vi "cRIO Open Module Detect_9104.vi"(8 "error in (no error)":errorcluster, 11 "RIO Device":string="RIO0") -> (0 "error out":errorcluster, 2 "slots":i32, 3 "Refnum out":refnum<k20>)   [LabVIEW 2015]
uses:
  <vilib>/FPGAPlugInAG/cRIO-9104/niLvFpga_Open_cRIO-9104.vi
  <vilib>/rvi/interface/common/dynamic/niFpgaDynamicAddResources.vi
  <vilib>/rvi/interface/nirviOpenFPGA/nirviOpenFPGA.xnode
  9104_ReadEEPROM.lvbitx
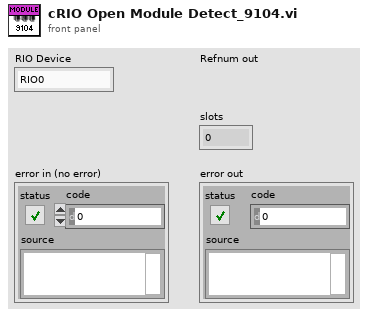
[diagram p1: front panel]
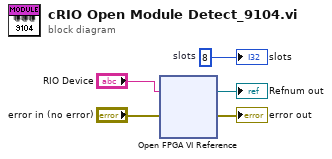
[diagram p0: block diagram]
diagram:
  w5 = 8  # slots
  n1 = xnode ("Open FPGA VI Reference")("error in"="error in (no error)", "resource name"="RIO Device") -> ("FPGA VI Reference Out"=→"Refnum out":refnum<k20>, "error out"=→"error out":errorcluster)
  "slots" <- w5
